vi "RunPreprocScript.vi"(8 "error in (no error)":errorcluster, 9 "Script":string, 10 "function name":string="exec_code", 11 "Python in":refnum<class "Python.lvclass">) -> (0 "error out":errorcluster, 2 "Out":string, 3 "Python out":refnum<class "Python.lvclass">)   [LabVIEW 2020, in "Python.lvclass"]
uses:
  Python.lvclass
  Python.lvclass/Python.ctl
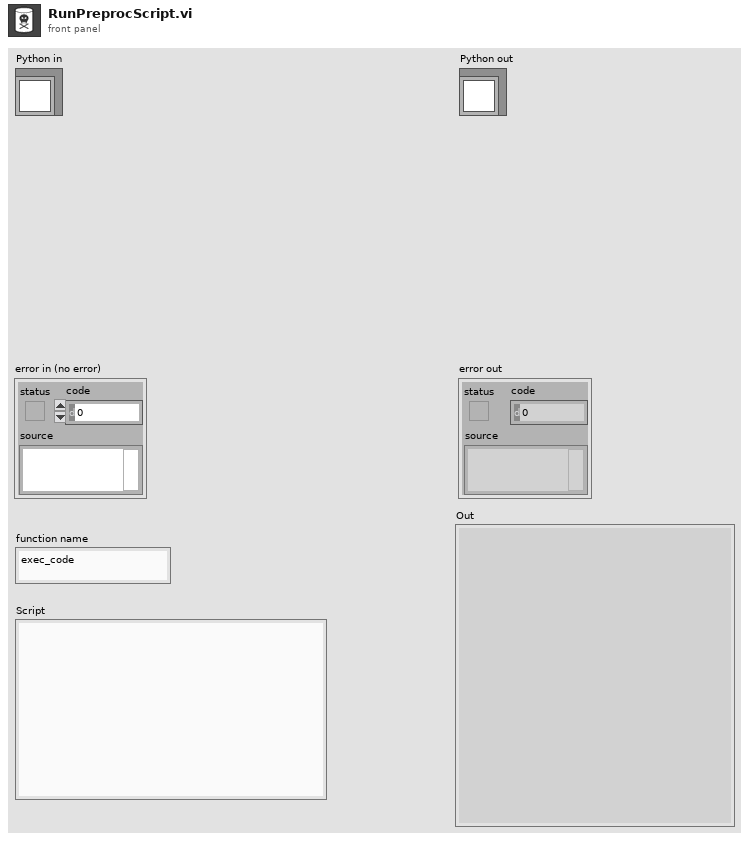
[diagram p1: front panel]
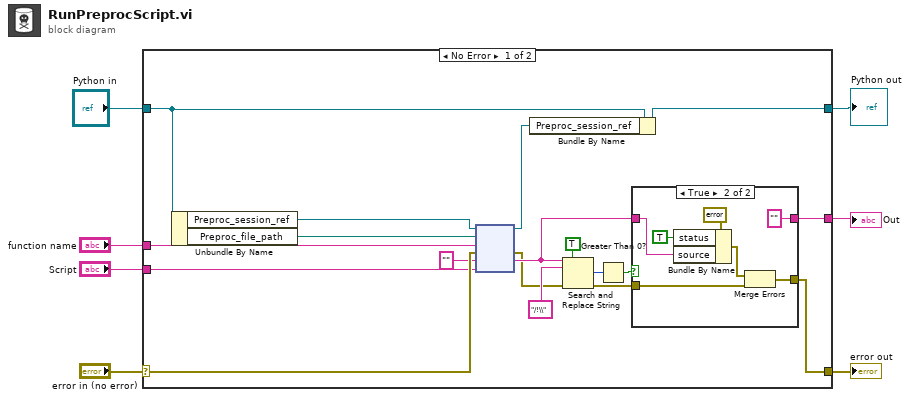
[diagram p0: block diagram]
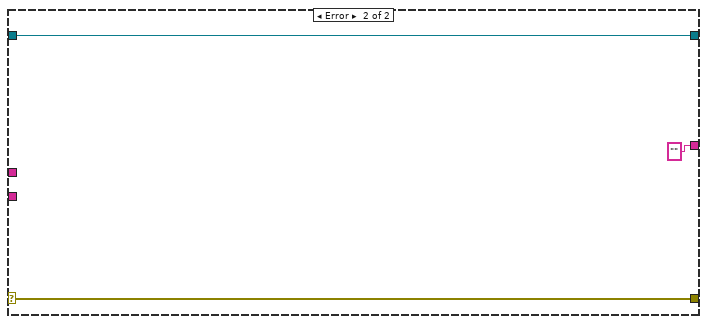
[diagram p3: hidden frame]
diagram:
  n1 = case shown="No Error" "error in (no error)" {
    selector: "error in (no error)" -> [w22 w37]
    tunnel: [w10 w37] -> w6
    tunnel: [w21 w36] -> w4
    tunnel: "Python in" -> [w25 w36]
    tunnel: "function name" -> [w19 _]
    tunnel: "Script" -> [w18 _]
    tunnel: [w11 ""] -> w1
    frame No Error {
      n2 = Unbundle By Name(w25) -> ("Preproc_session_ref"=w24:refnum<k35>, "Preproc_file_path"=w23:path)
      n3 = node(w24, w23, w19, w22, "", w18) -> (w20:refnum<k35>, w9:errorcluster, w12:string)  [unwired: 1 in, 2 out]
      n4 = Bundle By Name(cluster=w25, "Preproc_session_ref"=w20) -> (w21:refnum<class "Python.lvclass">)
      n5 = Search and Replace String(replace all?=TRUE ("replace all? (F)"), input string=w12, search string="/!\\", error in=w9) -> (number of replacements=w16:i32, error out=w17:errorcluster)  [unwired: 4 in, 2 out]
      n6 = Greater Than 0?(x=w16) -> (x > 0?=w15:bool)
      n7 = case shown="True" w15 {
        tunnel: w17 -> [w26 w31]
        tunnel: [w26 w30] -> w10
        tunnel: w12 -> [w27 w28]
        tunnel: [w27 ""] -> w11
        frame False {
        }
        frame True {
          n8 = Bundle By Name(cluster=errorcluster {"status"=FALSE, "code"=0, "source"=""} ("error constant"), "status"=TRUE, "source"=w28) -> (w32:errorcluster)
          n9 = Merge Errors(w32, w31) -> (w30:errorcluster)
        }
      }
    }
    frame Error {
    }
  }
  "error out" <- w6
  "Python out" <- w4
  "Out" <- w1
